vi "Set Database.vi"(8 "error in (no error)":errorcluster, 10 "Database":refnum<class "Database.lvclass">, 11 "ExcuseNotes in":refnum<class "ExcuseNotesHandler.lvclass">) -> (0 "error out":errorcluster, 3 "ExcuseNotes out":refnum<class "ExcuseNotesHandler.lvclass">)   [LabVIEW 2015, in "ExcuseNotesHandler.lvclass"]
uses:
  ExcuseNotesHandler.lvclass
  API/_Database/Database.lvclass
  ExcuseNotesHandler.lvclass/ExcuseNotesHandler.ctl
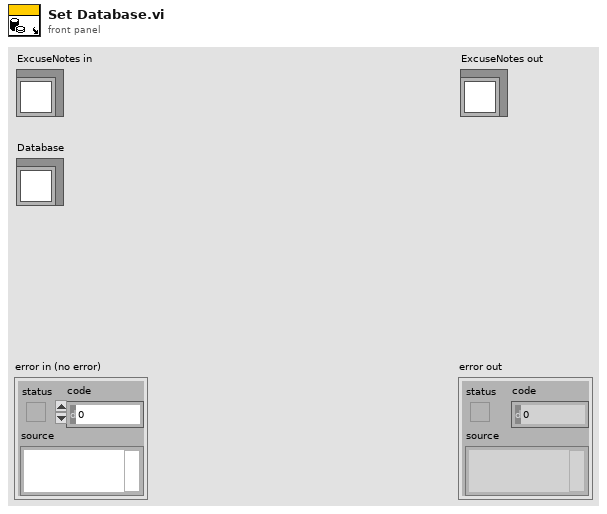
[diagram p1: front panel]
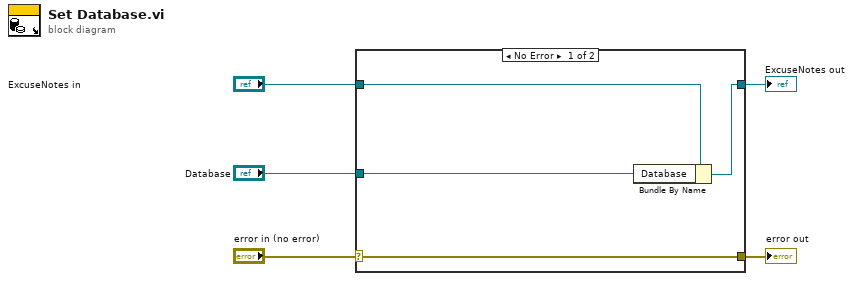
[diagram p0: block diagram]
diagram:
  n1 = case shown="No Error" "error in (no error)" {
    selector: "error in (no error)" -> [w9 w10]
    tunnel: [w9 w10] -> w4
    tunnel: [w7 w11] -> w2
    tunnel: "ExcuseNotes in" -> [w8 w11]
    tunnel: "Database" -> [w6 _]
    frame No Error {
      n2 = Bundle By Name(cluster=w8, "Database"=w6) -> (w7:refnum<class "ExcuseNotesHandler.lvclass">)
    }
    frame Error {
    }
  }
  "error out" <- w4
  "ExcuseNotes out" <- w2
